vi "sort_x.vi"(9 "y":dbl[](array[numeric]), 10 "x":dbl[](array[numeric])) -> (1 "sorted_y":dbl[](array[numeric]), 2 "sorted_x":dbl[](array[numeric]))   [LabVIEW 2017, in "tools.lvlib"]
uses:
  tools.lvlib
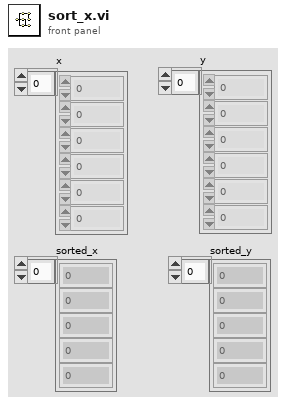
[diagram p1: front panel]
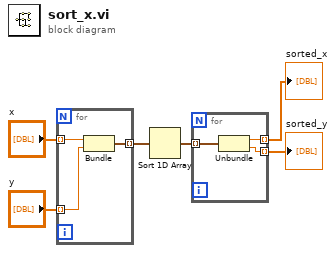
[diagram p0: block diagram]
diagram:
  n1 = for {
    tunnel: "x" -> [w9] mode=indexing
    tunnel: "y" -> [w8] mode=indexing
    tunnel: [w7] -> w4 mode=indexing
    n2 = Bundle("Numeric"=w9, "Numeric"=w8) -> (w7:cluster{"Numeric":dbl, "Numeric":dbl})  [unwired: 1 in]
  }
  n3 = Sort 1D Array(array=w4) -> (sorted array=w3:cluster{"Numeric":dbl, "Numeric":dbl}[])
  n4 = for {
    tunnel: w3 -> [w12] mode=indexing
    tunnel: [w11] -> w2 mode=indexing
    tunnel: [w10] -> w1 mode=indexing
    n5 = Unbundle(w12) -> ("Numeric"=w11:dbl, "Numeric"=w10:dbl)
  }
  "sorted_x" <- w2
  "sorted_y" <- w1
